vi "Inficon - Test connection.vi"(8 "Error In":errorcluster, 11 "COM in":refnum<visa-resource-name>) -> (0 "Error Out":errorcluster, 2 "Success?":bool, 3 "COM out":refnum<visa-resource-name>)   [LabVIEW 2014]
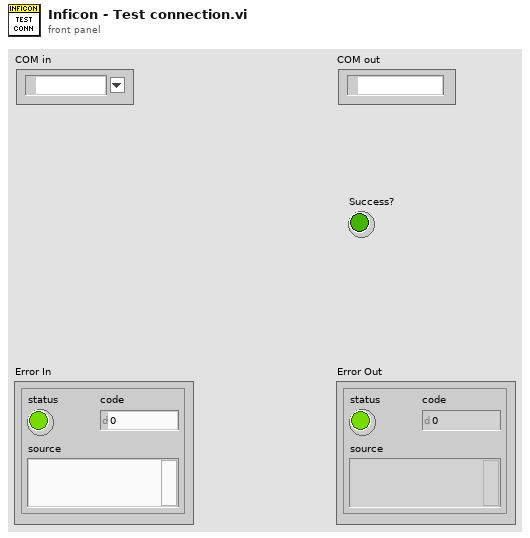
[diagram p1: front panel]
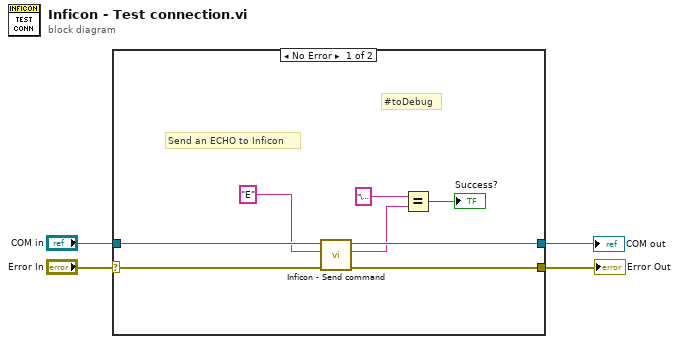
[diagram p0: block diagram]
diagram:
  n1 = case shown="No Error" "Error In" {
    selector: "Error In" -> [w12 w13]
    tunnel: [w11 w13] -> w3
    tunnel: "COM in" -> [w10 w14]
    tunnel: [w9 w14] -> w1
    frame No Error {
      # "#toDebug"
      # "Send an ECHO to Inficon"
      n2 = call "Inficon - Send command.vi"("Error In"=w12, "Command"="E", "COM in"=w10) -> ("Error Out"=w11:errorcluster, "Output"=w7:string, "COM out"=w9:refnum<visa-resource-name>)  [unwired: 6 in]
      n3 = Equal?(x="\u0006", y=w7) -> (x = y?=→"Success?":bool)
    }
    frame Error {
    }
  }
  "Error Out" <- w3
  "COM out" <- w1
